vi "sub_joystick-data-conv.vi"(11 "joystick info-in":T1) -> (3 "opval":cluster{dbl, dbl} {"?" format="%-1.1f"; "?" format="%-1.1f"})   [LabVIEW 2019]
panel:
  out "x*y":dbl
  out "x+y":dbl
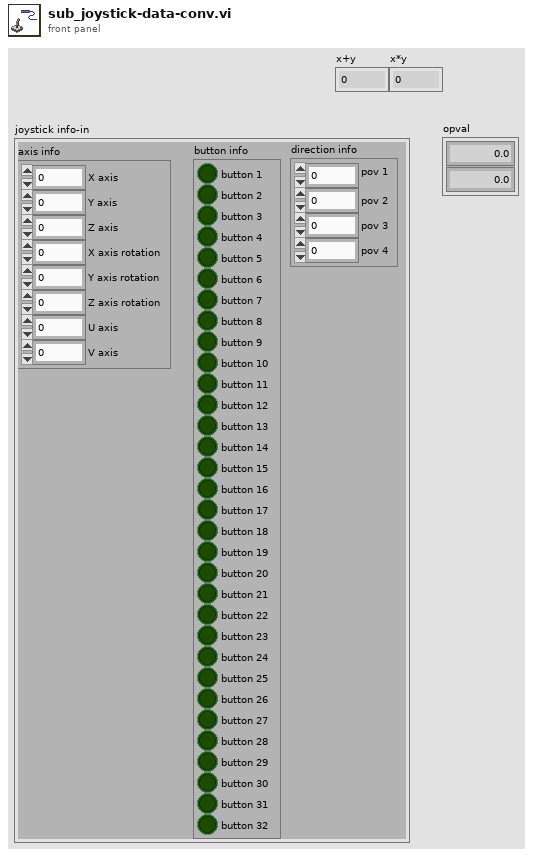
[diagram p1: front panel]
types:
  T1 = cluster{"axis info":cluster{"X axis":i32, "Y axis":i32, "Z axis":i32, "X axis rotation":i32, "Y axis rotation":i32, "Z axis rotation":i32, "U axis":i32, "V axis":i32}, "button info":cluster{"button 1":bool, "button 2":bool, "button 3":bool, "button 4":bool, "button 5":bool, "button 6":bool, "button 7":bool, "button 8":bool, "button 9":bool, "button 10":bool, "button 11":bool, "button 12":bool, "button 13":bool, "button 14":bool, "button 15":bool, "button 16":bool, "button 17":bool, "button 18":bool, "button 19":bool, "button 20":bool, "button 21":bool, "button 22":bool, "button 23":bool, "button 24":bool, "button 25":bool, "button 26":bool, "button 27":bool, "button 28":bool, "button 29":bool, "button 30":bool, "button 31":bool, "button 32":bool}, "direction info":cluster{"pov 1":i32, "pov 2":i32, "pov 3":i32, "pov 4":i32}}
  T2 = typedef "system_hw.ctl" = cluster{"AGV":enum16{"none", "ERP42", "ERP42mini", "Scout", "Ycar"}, "Lidar 1":enum16{"none", "VLP16", "TIM571", "RPLidar A2", "RPLidar A3"}, "Lidar 2":enum16{"none", "VLP16", "TIM571", "RPLidar A2", "RPLidar A3"}, "GPS":enum16{"none", "F9P", "M8P", "PwrPak7", "19X HVS"}, "Camera":enum16{"none", "C920", "C922", "GT1290C", "MS LifeCam"}, "Joystick":enum16{"none", "joystick"}}
  T3 = enum16{"none", "ERP42", "ERP42mini", "Scout", "Ycar"}
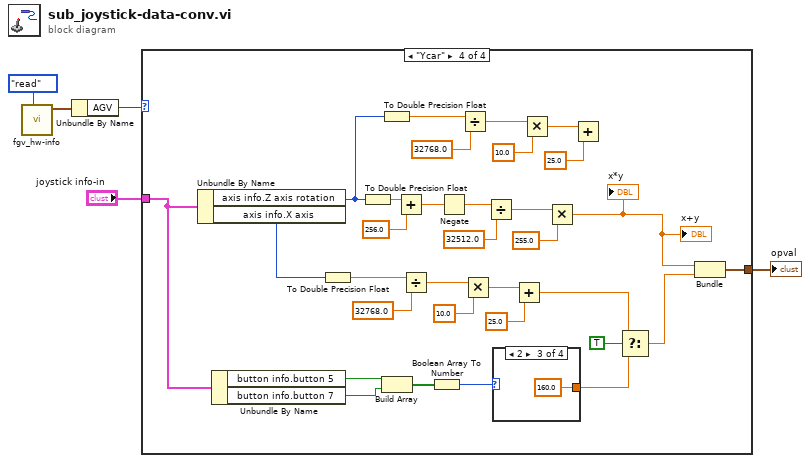
[diagram p0: block diagram]
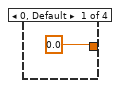
[diagram p5: hidden frame]
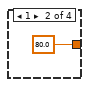
[diagram p6: hidden frame]
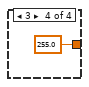
[diagram p7: hidden frame]
diagram:
  n1 = call "fgv_hw-info.vi"("cmd"=enum16{"write", "read"}."read") -> ("HW info out"=w2:T2)  [unwired: 10 in]
  n2 = Unbundle By Name(w2) -> ("AGV"=w1:T3)
  n3 = case shown="\"Ycar\"" w1 {
    tunnel: [_ _ _ w37] -> w5
    tunnel: "joystick info-in" -> [_ _ _ w16]
    frame "ERP42", Default {
    }
    frame "ERP42mini" {
    }
    frame "Scout" {
    }
    frame "Ycar" {
      n4 = Unbundle By Name(w16) -> ("axis info.Z axis rotation"=w7:i32, "axis info.X axis"=w29:i32)
      n5 = Unbundle By Name(w16) -> ("button info.button 5"=w14:bool, "button info.button 7"=w15:bool)
      n6 = To Double Precision Float(number=w29) -> (double precision float=w23:dbl)
      n7 = To Double Precision Float(number=w7) -> (double precision float=w24:dbl)
      n8 = To Double Precision Float(number=w7) -> (double precision float=w22:dbl)
      n9 = Build Array(w14, w15) -> (w13:bool[])
      n10 = Add(x=w24, y=256.0) -> (x+y=w35:dbl)
      n11 = Divide(x=w23, y=32768.0) -> (x/y=w27:dbl)
      n12 = Boolean Array To Number(Boolean array=w13) -> (number=w12:u32)
      n13 = Negate(x=w35) -> (-x=w33:dbl)
      n14 = Divide(x=w22, y=32768.0) -> (x/y=w19:dbl)
      n15 = Multiply(x=w27, y=10.0) -> (x*y=w25:dbl)
      n16 = Divide(x=w33, y=32512.0) -> (x/y=w32:dbl)
      n17 = case shown="2" w12 {
        tunnel: [0.0 80.0 160.0 255.0] -> w10
        frame 0, Default {
        }
        frame 1 {
        }
        frame 2 {
        }
        frame 3 {
        }
      }
      n18 = Add(x=w25, y=25.0) -> (x+y=w11:dbl)
      n19 = Multiply(x=w19, y=10.0) -> (x*y=w21:dbl)
      n20 = Multiply(x=w32, y=255.0) -> (x*y=w6:dbl)
      "x+y" <- w6
      "x*y" <- w6
      n21 = Add(x=w21, y=25.0) -> ()  [unwired: 1 out]
      n22 = Select(t=w11, s=TRUE, f=w10) -> (s? t:f=w8:dbl)
      n23 = Bundle(w6, w8) -> (w37:cluster{dbl, dbl})  [unwired: 1 in]
    }
  }
  "opval" <- w5
